vi "WIP lock-in auto-adjust sensitivty.vi"() -> ()   [LabVIEW 2017]
uses:
  Lockin SR830.lvclass
panel:
  out "Lockin SR830.lvclass out":refnum<class "Lockin SR830.lvclass">
  out "error out":errorcluster
  in  "error in (no error)":errorcluster
  in  "Lockin SR830.lvclass In":refnum<class "Lockin SR830.lvclass">
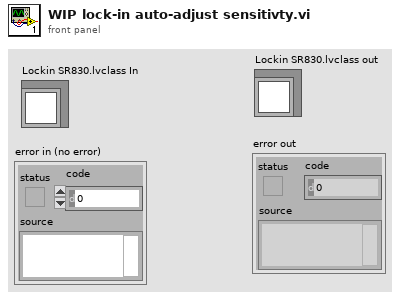
[diagram p1: front panel]
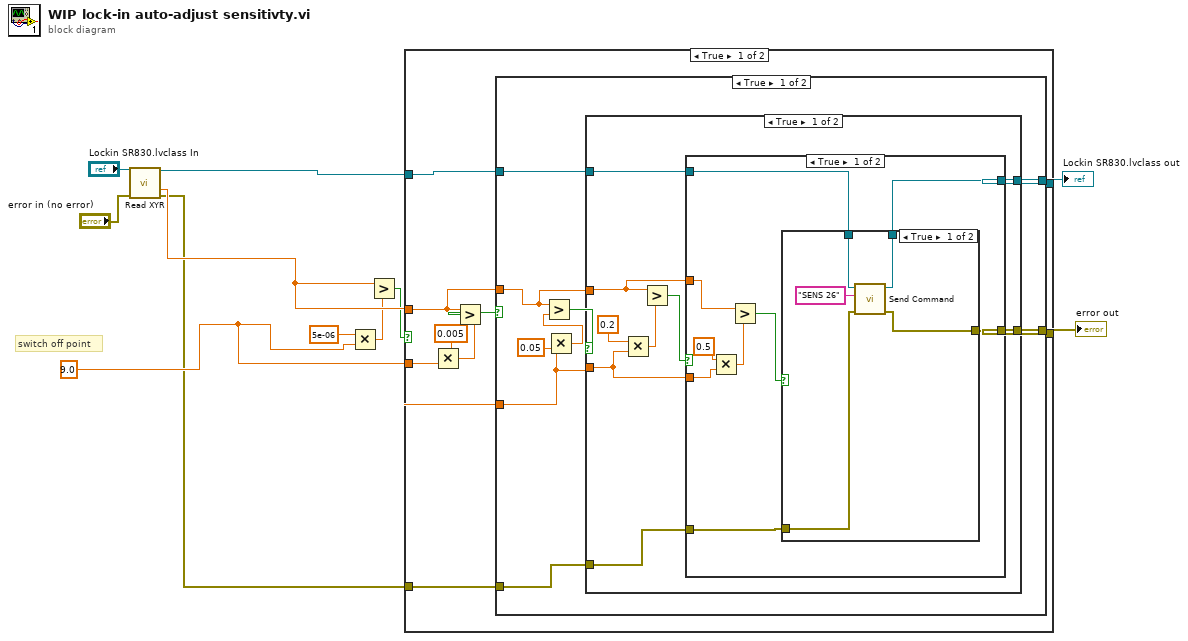
[diagram p0: block diagram]
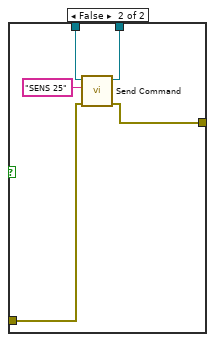
[diagram p2: hidden frame]
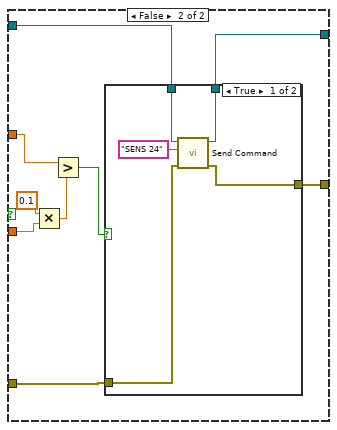
[diagram p3: hidden frame]
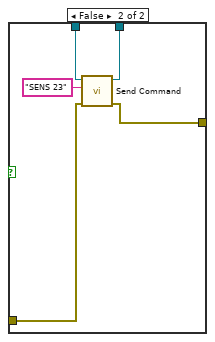
[diagram p4: hidden frame]
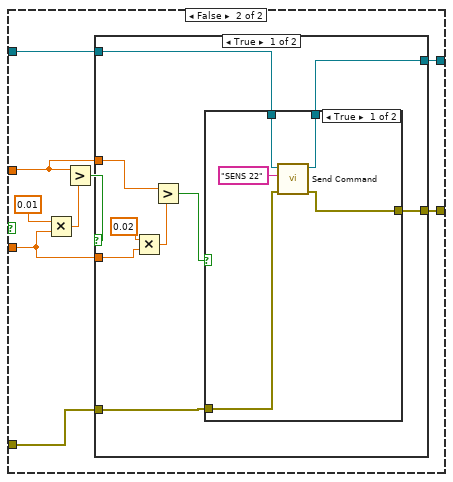
[diagram p5: hidden frame]
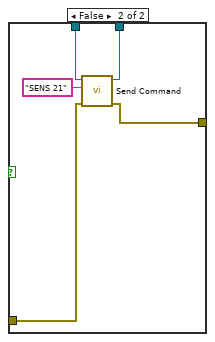
[diagram p6: hidden frame]
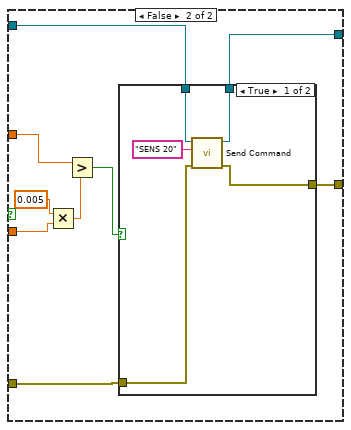
[diagram p7: hidden frame]
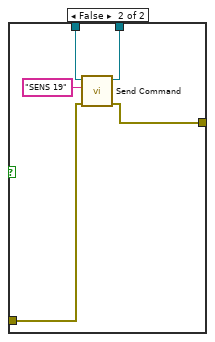
[diagram p8: hidden frame]
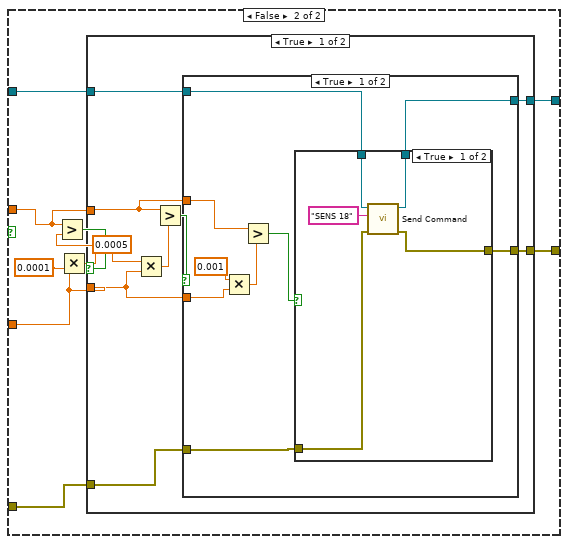
[diagram p9: hidden frame]
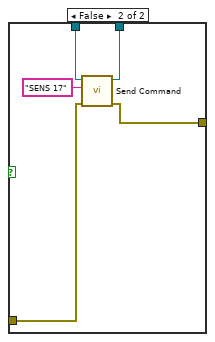
[diagram p10: hidden frame]
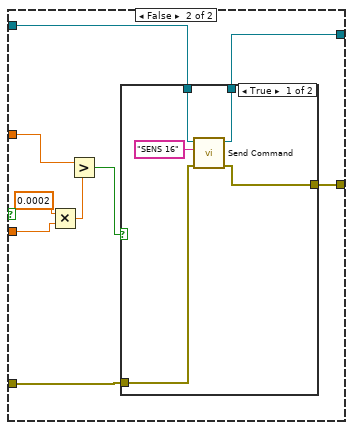
[diagram p11: hidden frame]
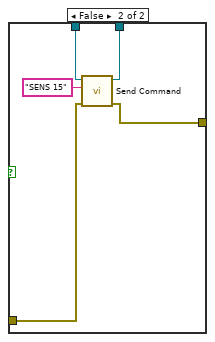
[diagram p12: hidden frame]
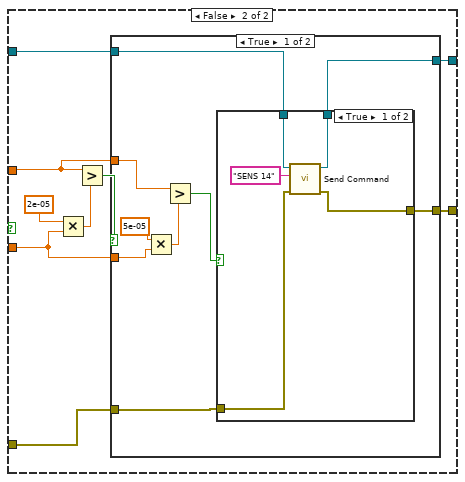
[diagram p13: hidden frame]
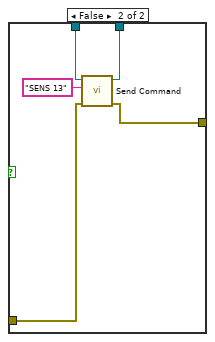
[diagram p14: hidden frame]
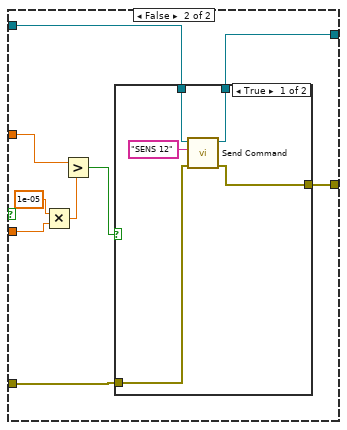
[diagram p15: hidden frame]
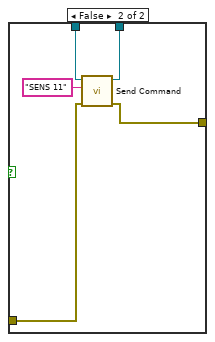
[diagram p16: hidden frame]
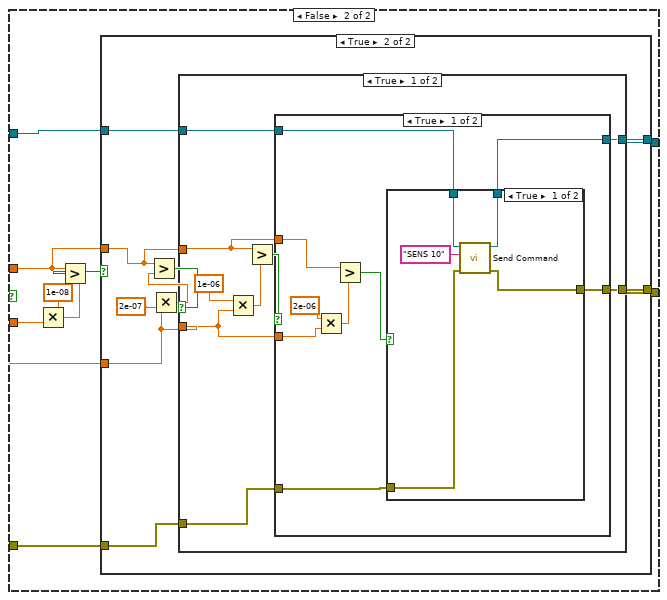
[diagram p17: hidden frame]
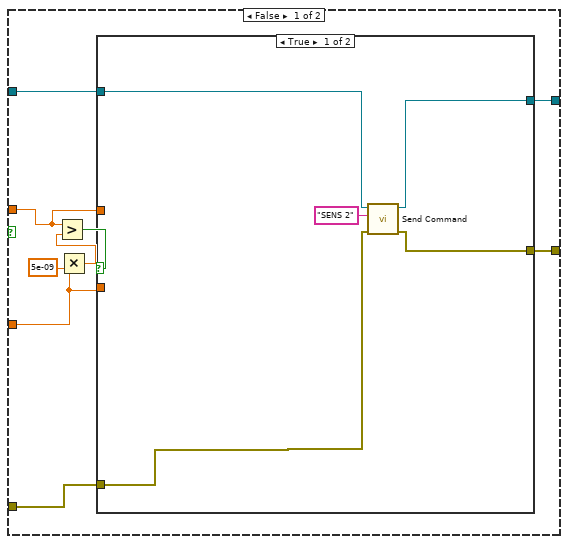
[diagram p18: hidden frame]
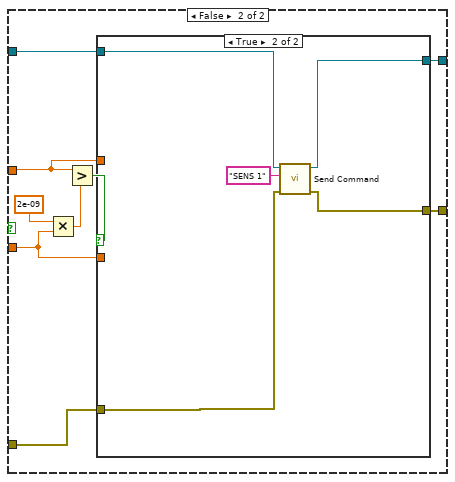
[diagram p19: hidden frame]
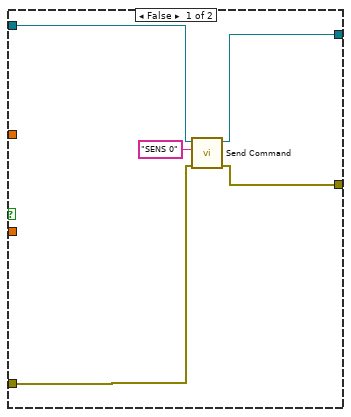
[diagram p20: hidden frame]
diagram:
  w9 = 9.0
  # "switch off point"
  n1 = call "Read XYR.vi"("Lockin SR830 in"="Lockin SR830.lvclass In", "error in (no error)"="error in (no error)") -> ("Lockin SR830 out"=w7:refnum<class "Lockin SR830.lvclass">, "R"=w8:dbl, "error out"=w5:errorcluster)  [unwired: 9 in, 2 out]
  n2 = Multiply(x=5e-06, y=w9) -> (x*y=w3:dbl)
  n3 = Greater?(x=w8, y=w3) -> (0:w1:bool)
  n4 = case shown="True" w1 {
    tunnel: w8 -> [w17 w232]
    tunnel: w9 -> [w16 w231]
    tunnel: w7 -> [w15 w230]
    tunnel: [w14 w229] -> w6
    tunnel: w5 -> [w13 w228]
    tunnel: [w12 w227] -> w4
    frame True {
      n5 = Multiply(x=0.005, y=w16) -> (x*y=w20:dbl)
      n6 = Greater?(x=w17, y=w20) -> (0:w19:bool)
      n7 = case shown="True" w19 {
        tunnel: w17 -> [w25 w128]
        tunnel: w16 -> [w26 w129]
        tunnel: w15 -> [w24 w127]
        tunnel: [w23 w126] -> w14
        tunnel: w13 -> [w22 w125]
        tunnel: [w21 w124] -> w12
        frame True {
          n8 = Multiply(x=w26, y=0.05) -> (x*y=w29:dbl)
          n9 = Greater?(x=w25, y=w29) -> (0:w27:bool)
          n10 = case shown="True" w27 {
            tunnel: w26 -> [w35 w82]
            tunnel: w25 -> [w34 w81]
            tunnel: w24 -> [w33 w80]
            tunnel: [w32 w79] -> w23
            tunnel: w22 -> [w31 w78]
            tunnel: [w30 w77] -> w21
            frame True {
              n11 = Multiply(x=0.2, y=w35) -> (x*y=w38:dbl)
              n12 = Greater?(x=w34, y=w38) -> (0:w36:bool)
              n13 = case shown="True" w36 {
                tunnel: w35 -> [w46 w65]
                tunnel: w34 -> [w44 w63]
                tunnel: w33 -> [w42 w61]
                tunnel: [w41 w60] -> w32
                tunnel: w31 -> [w39 w58]
                tunnel: [w40 w59] -> w30
                frame True {
                  n14 = Multiply(x=0.5, y=w46) -> (x*y=w47:dbl)
                  n15 = Greater?(x=w44, y=w47) -> (0:w43:bool)
                  n16 = case shown="True" w43 {
                    tunnel: w42 -> [w52 w57]
                    tunnel: [w51 w56] -> w41
                    tunnel: [w50 w55] -> w40
                    tunnel: w39 -> [w49 w54]
                    frame True {
                      n17 = call "Send Command.vi"("error in (no error)"=w49, "Command String"="SENS 26", "Lockin SR830.lvclass In"=w52) -> ("error out"=w50:errorcluster, "Lockin SR830.lvclass out"=w51:refnum<class "Lockin SR830.lvclass">)  [unwired: 7 in]
                    }
                    frame False {
                      n18 = call "Send Command.vi"("error in (no error)"=w54, "Command String"="SENS 25", "Lockin SR830.lvclass In"=w57) -> ("error out"=w55:errorcluster, "Lockin SR830.lvclass out"=w56:refnum<class "Lockin SR830.lvclass">)  [unwired: 7 in]
                    }
                  }
                }
                frame False {
                  n19 = Multiply(x=0.1, y=w65) -> (x*y=w66:dbl)
                  n20 = Greater?(x=w63, y=w66) -> (0:w62:bool)
                  n21 = case shown="True" w62 {
                    tunnel: w61 -> [w71 w76]
                    tunnel: [w70 w75] -> w60
                    tunnel: [w69 w74] -> w59
                    tunnel: w58 -> [w68 w73]
                    frame True {
                      n22 = call "Send Command.vi"("error in (no error)"=w68, "Command String"="SENS 24", "Lockin SR830.lvclass In"=w71) -> ("error out"=w69:errorcluster, "Lockin SR830.lvclass out"=w70:refnum<class "Lockin SR830.lvclass">)  [unwired: 7 in]
                    }
                    frame False {
                      n23 = call "Send Command.vi"("error in (no error)"=w73, "Command String"="SENS 23", "Lockin SR830.lvclass In"=w76) -> ("error out"=w74:errorcluster, "Lockin SR830.lvclass out"=w75:refnum<class "Lockin SR830.lvclass">)  [unwired: 7 in]
                    }
                  }
                }
              }
            }
            frame False {
              n24 = Multiply(x=0.01, y=w82) -> (x*y=w85:dbl)
              n25 = Greater?(x=w81, y=w85) -> (0:w83:bool)
              n26 = case shown="True" w83 {
                tunnel: w82 -> [w93 w112]
                tunnel: w81 -> [w91 w110]
                tunnel: w80 -> [w89 w108]
                tunnel: [w88 w107] -> w79
                tunnel: w78 -> [w86 w105]
                tunnel: [w87 w106] -> w77
                frame True {
                  n27 = Multiply(x=0.02, y=w93) -> (x*y=w94:dbl)
                  n28 = Greater?(x=w91, y=w94) -> (0:w90:bool)
                  n29 = case shown="True" w90 {
                    tunnel: w89 -> [w99 w104]
                    tunnel: [w98 w103] -> w88
                    tunnel: [w97 w102] -> w87
                    tunnel: w86 -> [w96 w101]
                    frame True {
                      n30 = call "Send Command.vi"("error in (no error)"=w96, "Command String"="SENS 22", "Lockin SR830.lvclass In"=w99) -> ("error out"=w97:errorcluster, "Lockin SR830.lvclass out"=w98:refnum<class "Lockin SR830.lvclass">)  [unwired: 7 in]
                    }
                    frame False {
                      n31 = call "Send Command.vi"("error in (no error)"=w101, "Command String"="SENS 21", "Lockin SR830.lvclass In"=w104) -> ("error out"=w102:errorcluster, "Lockin SR830.lvclass out"=w103:refnum<class "Lockin SR830.lvclass">)  [unwired: 7 in]
                    }
                  }
                }
                frame False {
                  n32 = Multiply(x=0.005, y=w112) -> (x*y=w113:dbl)
                  n33 = Greater?(x=w110, y=w113) -> (0:w109:bool)
                  n34 = case shown="True" w109 {
                    tunnel: w108 -> [w118 w123]
                    tunnel: [w117 w122] -> w107
                    tunnel: [w116 w121] -> w106
                    tunnel: w105 -> [w115 w120]
                    frame True {
                      n35 = call "Send Command.vi"("error in (no error)"=w115, "Command String"="SENS 20", "Lockin SR830.lvclass In"=w118) -> ("error out"=w116:errorcluster, "Lockin SR830.lvclass out"=w117:refnum<class "Lockin SR830.lvclass">)  [unwired: 7 in]
                    }
                    frame False {
                      n36 = call "Send Command.vi"("error in (no error)"=w120, "Command String"="SENS 19", "Lockin SR830.lvclass In"=w123) -> ("error out"=w121:errorcluster, "Lockin SR830.lvclass out"=w122:refnum<class "Lockin SR830.lvclass">)  [unwired: 7 in]
                    }
                  }
                }
              }
            }
          }
        }
        frame False {
          n37 = Multiply(x=w129, y=0.0001) -> (x*y=w132:dbl)
          n38 = Greater?(x=w128, y=w132) -> (0:w130:bool)
          n39 = case shown="True" w130 {
            tunnel: w129 -> [w138 w185]
            tunnel: w128 -> [w137 w184]
            tunnel: w127 -> [w136 w183]
            tunnel: [w135 w182] -> w126
            tunnel: w125 -> [w134 w181]
            tunnel: [w133 w180] -> w124
            frame True {
              n40 = Multiply(x=0.0005, y=w138) -> (x*y=w141:dbl)
              n41 = Greater?(x=w137, y=w141) -> (0:w139:bool)
              n42 = case shown="True" w139 {
                tunnel: w138 -> [w149 w168]
                tunnel: w137 -> [w147 w166]
                tunnel: w136 -> [w145 w164]
                tunnel: [w144 w163] -> w135
                tunnel: w134 -> [w142 w161]
                tunnel: [w143 w162] -> w133
                frame True {
                  n43 = Multiply(x=0.001, y=w149) -> (x*y=w150:dbl)
                  n44 = Greater?(x=w147, y=w150) -> (0:w146:bool)
                  n45 = case shown="True" w146 {
                    tunnel: w145 -> [w155 w160]
                    tunnel: [w154 w159] -> w144
                    tunnel: [w153 w158] -> w143
                    tunnel: w142 -> [w152 w157]
                    frame True {
                      n46 = call "Send Command.vi"("error in (no error)"=w152, "Command String"="SENS 18", "Lockin SR830.lvclass In"=w155) -> ("error out"=w153:errorcluster, "Lockin SR830.lvclass out"=w154:refnum<class "Lockin SR830.lvclass">)  [unwired: 7 in]
                    }
                    frame False {
                      n47 = call "Send Command.vi"("error in (no error)"=w157, "Command String"="SENS 17", "Lockin SR830.lvclass In"=w160) -> ("error out"=w158:errorcluster, "Lockin SR830.lvclass out"=w159:refnum<class "Lockin SR830.lvclass">)  [unwired: 7 in]
                    }
                  }
                }
                frame False {
                  n48 = Multiply(x=0.0002, y=w168) -> (x*y=w169:dbl)
                  n49 = Greater?(x=w166, y=w169) -> (0:w165:bool)
                  n50 = case shown="True" w165 {
                    tunnel: w164 -> [w174 w179]
                    tunnel: [w173 w178] -> w163
                    tunnel: [w172 w177] -> w162
                    tunnel: w161 -> [w171 w176]
                    frame True {
                      n51 = call "Send Command.vi"("error in (no error)"=w171, "Command String"="SENS 16", "Lockin SR830.lvclass In"=w174) -> ("error out"=w172:errorcluster, "Lockin SR830.lvclass out"=w173:refnum<class "Lockin SR830.lvclass">)  [unwired: 7 in]
                    }
                    frame False {
                      n52 = call "Send Command.vi"("error in (no error)"=w176, "Command String"="SENS 15", "Lockin SR830.lvclass In"=w179) -> ("error out"=w177:errorcluster, "Lockin SR830.lvclass out"=w178:refnum<class "Lockin SR830.lvclass">)  [unwired: 7 in]
                    }
                  }
                }
              }
            }
            frame False {
              n53 = Multiply(x=2e-05, y=w185) -> (x*y=w188:dbl)
              n54 = Greater?(x=w184, y=w188) -> (0:w186:bool)
              n55 = case shown="True" w186 {
                tunnel: w185 -> [w196 w215]
                tunnel: w184 -> [w194 w213]
                tunnel: w183 -> [w192 w211]
                tunnel: [w191 w210] -> w182
                tunnel: w181 -> [w189 w208]
                tunnel: [w190 w209] -> w180
                frame True {
                  n56 = Multiply(x=5e-05, y=w196) -> (x*y=w197:dbl)
                  n57 = Greater?(x=w194, y=w197) -> (0:w193:bool)
                  n58 = case shown="True" w193 {
                    tunnel: w192 -> [w202 w207]
                    tunnel: [w201 w206] -> w191
                    tunnel: [w200 w205] -> w190
                    tunnel: w189 -> [w199 w204]
                    frame True {
                      n59 = call "Send Command.vi"("error in (no error)"=w199, "Command String"="SENS 14", "Lockin SR830.lvclass In"=w202) -> ("error out"=w200:errorcluster, "Lockin SR830.lvclass out"=w201:refnum<class "Lockin SR830.lvclass">)  [unwired: 7 in]
                    }
                    frame False {
                      n60 = call "Send Command.vi"("error in (no error)"=w204, "Command String"="SENS 13", "Lockin SR830.lvclass In"=w207) -> ("error out"=w205:errorcluster, "Lockin SR830.lvclass out"=w206:refnum<class "Lockin SR830.lvclass">)  [unwired: 7 in]
                    }
                  }
                }
                frame False {
                  n61 = Multiply(x=1e-05, y=w215) -> (x*y=w216:dbl)
                  n62 = Greater?(x=w213, y=w216) -> (0:w212:bool)
                  n63 = case shown="True" w212 {
                    tunnel: w211 -> [w221 w226]
                    tunnel: [w220 w225] -> w210
                    tunnel: [w219 w224] -> w209
                    tunnel: w208 -> [w218 w223]
                    frame True {
                      n64 = call "Send Command.vi"("error in (no error)"=w218, "Command String"="SENS 12", "Lockin SR830.lvclass In"=w221) -> ("error out"=w219:errorcluster, "Lockin SR830.lvclass out"=w220:refnum<class "Lockin SR830.lvclass">)  [unwired: 7 in]
                    }
                    frame False {
                      n65 = call "Send Command.vi"("error in (no error)"=w223, "Command String"="SENS 11", "Lockin SR830.lvclass In"=w226) -> ("error out"=w224:errorcluster, "Lockin SR830.lvclass out"=w225:refnum<class "Lockin SR830.lvclass">)  [unwired: 7 in]
                    }
                  }
                }
              }
            }
          }
        }
      }
    }
    frame False {
      n66 = Multiply(x=1e-08, y=w231) -> (x*y=w235:dbl)
      n67 = Greater?(x=w232, y=w235) -> (0:w234:bool)
      n68 = case shown="True" w234 {
        tunnel: w232 -> [w240 w273]
        tunnel: w231 -> [w241 w274]
        tunnel: w230 -> [w239 w272]
        tunnel: [w238 w271] -> w229
        tunnel: w228 -> [w237 w270]
        tunnel: [w236 w269] -> w227
        frame False {
          n69 = Multiply(x=w241, y=5e-09) -> (x*y=w244:dbl)
          n70 = Greater?(x=w240, y=w244) -> (0:w242:bool)
          n71 = case shown="True" w242 {
            tunnel: w241 -> [_ w255]
            tunnel: w240 -> [_ w254]
            tunnel: w239 -> [w249 w253]
            tunnel: [w248 w252] -> w238
            tunnel: w237 -> [w247 w251]
            tunnel: [w246 w250] -> w236
            frame True {
              n72 = call "Send Command.vi"("error in (no error)"=w247, "Command String"="SENS 2", "Lockin SR830.lvclass In"=w249) -> ("error out"=w246:errorcluster, "Lockin SR830.lvclass out"=w248:refnum<class "Lockin SR830.lvclass">)  [unwired: 7 in]
            }
            frame False {
              n73 = Multiply(x=2e-09, y=w255) -> (x*y=w258:dbl)
              n74 = Greater?(x=w254, y=w258) -> (0:w256:bool)
              n75 = case shown="True" w256 {
                tunnel: w255 -> [_ _]
                tunnel: w254 -> [_ _]
                tunnel: w253 -> [w263 w268]
                tunnel: [w262 w267] -> w252
                tunnel: w251 -> [w260 w265]
                tunnel: [w261 w266] -> w250
                frame False {
                  n76 = call "Send Command.vi"("error in (no error)"=w260, "Command String"="SENS 0", "Lockin SR830.lvclass In"=w263) -> ("error out"=w261:errorcluster, "Lockin SR830.lvclass out"=w262:refnum<class "Lockin SR830.lvclass">)  [unwired: 7 in]
                }
                frame True {
                  n77 = call "Send Command.vi"("error in (no error)"=w265, "Command String"="SENS 1", "Lockin SR830.lvclass In"=w268) -> ("error out"=w266:errorcluster, "Lockin SR830.lvclass out"=w267:refnum<class "Lockin SR830.lvclass">)  [unwired: 7 in]
                }
              }
            }
          }
        }
        frame True {
          n78 = Multiply(x=w274, y=2e-07) -> (x*y=w277:dbl)
          n79 = Greater?(x=w273, y=w277) -> (0:w275:bool)
          n80 = case shown="True" w275 {
            tunnel: w274 -> [w283 w330]
            tunnel: w273 -> [w282 w329]
            tunnel: w272 -> [w281 w328]
            tunnel: [w280 w327] -> w271
            tunnel: w270 -> [w279 w326]
            tunnel: [w278 w325] -> w269
            frame True {
              n81 = Multiply(x=1e-06, y=w283) -> (x*y=w286:dbl)
              n82 = Greater?(x=w282, y=w286) -> (0:w284:bool)
              n83 = case shown="True" w284 {
                tunnel: w283 -> [w294 w313]
                tunnel: w282 -> [w292 w311]
                tunnel: w281 -> [w290 w309]
                tunnel: [w289 w308] -> w280
                tunnel: w279 -> [w287 w306]
                tunnel: [w288 w307] -> w278
                frame True {
                  n84 = Multiply(x=2e-06, y=w294) -> (x*y=w295:dbl)
                  n85 = Greater?(x=w292, y=w295) -> (0:w291:bool)
                  n86 = case shown="True" w291 {
                    tunnel: w290 -> [w300 w305]
                    tunnel: [w299 w304] -> w289
                    tunnel: [w298 w303] -> w288
                    tunnel: w287 -> [w297 w302]
                    frame True {
                      n87 = call "Send Command.vi"("error in (no error)"=w297, "Command String"="SENS 10", "Lockin SR830.lvclass In"=w300) -> ("error out"=w298:errorcluster, "Lockin SR830.lvclass out"=w299:refnum<class "Lockin SR830.lvclass">)  [unwired: 7 in]
                    }
                    frame False {
                      n88 = call "Send Command.vi"("error in (no error)"=w302, "Command String"="SENS 9", "Lockin SR830.lvclass In"=w305) -> ("error out"=w303:errorcluster, "Lockin SR830.lvclass out"=w304:refnum<class "Lockin SR830.lvclass">)  [unwired: 7 in]
                    }
                  }
                }
                frame False {
                  n89 = Multiply(x=5e-07, y=w313) -> (x*y=w314:dbl)
                  n90 = Greater?(x=w311, y=w314) -> (0:w310:bool)
                  n91 = case shown="True" w310 {
                    tunnel: w309 -> [w319 w324]
                    tunnel: [w318 w323] -> w308
                    tunnel: [w317 w322] -> w307
                    tunnel: w306 -> [w316 w321]
                    frame True {
                      n92 = call "Send Command.vi"("error in (no error)"=w316, "Command String"="SENS 8", "Lockin SR830.lvclass In"=w319) -> ("error out"=w317:errorcluster, "Lockin SR830.lvclass out"=w318:refnum<class "Lockin SR830.lvclass">)  [unwired: 7 in]
                    }
                    frame False {
                      n93 = call "Send Command.vi"("error in (no error)"=w321, "Command String"="SENS 7", "Lockin SR830.lvclass In"=w324) -> ("error out"=w322:errorcluster, "Lockin SR830.lvclass out"=w323:refnum<class "Lockin SR830.lvclass">)  [unwired: 7 in]
                    }
                  }
                }
              }
            }
            frame False {
              n94 = Multiply(x=5e-08, y=w330) -> (x*y=w333:dbl)
              n95 = Greater?(x=w329, y=w333) -> (0:w331:bool)
              n96 = case shown="True" w331 {
                tunnel: w330 -> [w341 w360]
                tunnel: w329 -> [w339 w358]
                tunnel: w328 -> [w337 w356]
                tunnel: [w336 w355] -> w327
                tunnel: w326 -> [w334 w353]
                tunnel: [w335 w354] -> w325
                frame True {
                  n97 = Multiply(x=1e-07, y=w341) -> (x*y=w342:dbl)
                  n98 = Greater?(x=w339, y=w342) -> (0:w338:bool)
                  n99 = case shown="True" w338 {
                    tunnel: w337 -> [w347 w352]
                    tunnel: [w346 w351] -> w336
                    tunnel: [w345 w350] -> w335
                    tunnel: w334 -> [w344 w349]
                    frame True {
                      n100 = call "Send Command.vi"("error in (no error)"=w344, "Command String"="SENS 6", "Lockin SR830.lvclass In"=w347) -> ("error out"=w345:errorcluster, "Lockin SR830.lvclass out"=w346:refnum<class "Lockin SR830.lvclass">)  [unwired: 7 in]
                    }
                    frame False {
                      n101 = call "Send Command.vi"("error in (no error)"=w349, "Command String"="SENS 5", "Lockin SR830.lvclass In"=w352) -> ("error out"=w350:errorcluster, "Lockin SR830.lvclass out"=w351:refnum<class "Lockin SR830.lvclass">)  [unwired: 7 in]
                    }
                  }
                }
                frame False {
                  n102 = Multiply(x=2e-08, y=w360) -> (x*y=w361:dbl)
                  n103 = Greater?(x=w358, y=w361) -> (0:w357:bool)
                  n104 = case shown="True" w357 {
                    tunnel: w356 -> [w366 w371]
                    tunnel: [w365 w370] -> w355
                    tunnel: [w364 w369] -> w354
                    tunnel: w353 -> [w363 w368]
                    frame True {
                      n105 = call "Send Command.vi"("error in (no error)"=w363, "Command String"="SENS 4", "Lockin SR830.lvclass In"=w366) -> ("error out"=w364:errorcluster, "Lockin SR830.lvclass out"=w365:refnum<class "Lockin SR830.lvclass">)  [unwired: 7 in]
                    }
                    frame False {
                      n106 = call "Send Command.vi"("error in (no error)"=w368, "Command String"="SENS 3", "Lockin SR830.lvclass In"=w371) -> ("error out"=w369:errorcluster, "Lockin SR830.lvclass out"=w370:refnum<class "Lockin SR830.lvclass">)  [unwired: 7 in]
                    }
                  }
                }
              }
            }
          }
        }
      }
    }
  }
  "error out" <- w4
  "Lockin SR830.lvclass out" <- w6
